vi "Smp_Data_transfer.vi"(0 "Connection ID":T1, 5 "SaveFilePath":path caption="Temp file path", 7 "Source file path":string, 9 "Read point":i32=256000, 11 "error in (no error)":errorcluster) -> (3 "Error Code":i16, 4 "Connection ID Out":T1, 6 "SaveFilePath.ref":path caption="Temp file path.ref", 10 "Stop":bool, 15 "error out":errorcluster)   [LabVIEW 2017]
uses:
  Driver/ConnectionID.ctl
  GL860_Driver.lvlib
panel:
  out "Progress bar":u8(slide) max=100 scale=0.0..100.0
  in  "Stop":bool
  # "Now transferring data..."
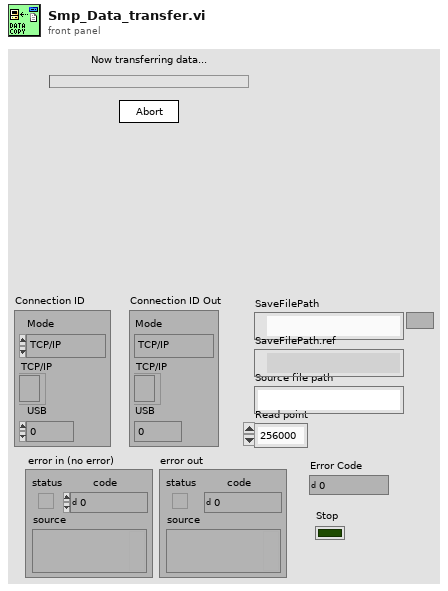
[diagram p1: front panel]
types:
  T1 = typedef "ConnectionID.ctl" = cluster{"Mode":enum16{"TCP/IP", "USB"}, "TCP/IP":refnum<k5>, "USB":i32}
  T2 = enum16{"open", "replace", "create", "open or create", "replace or create", "replace or create with confirmation"}
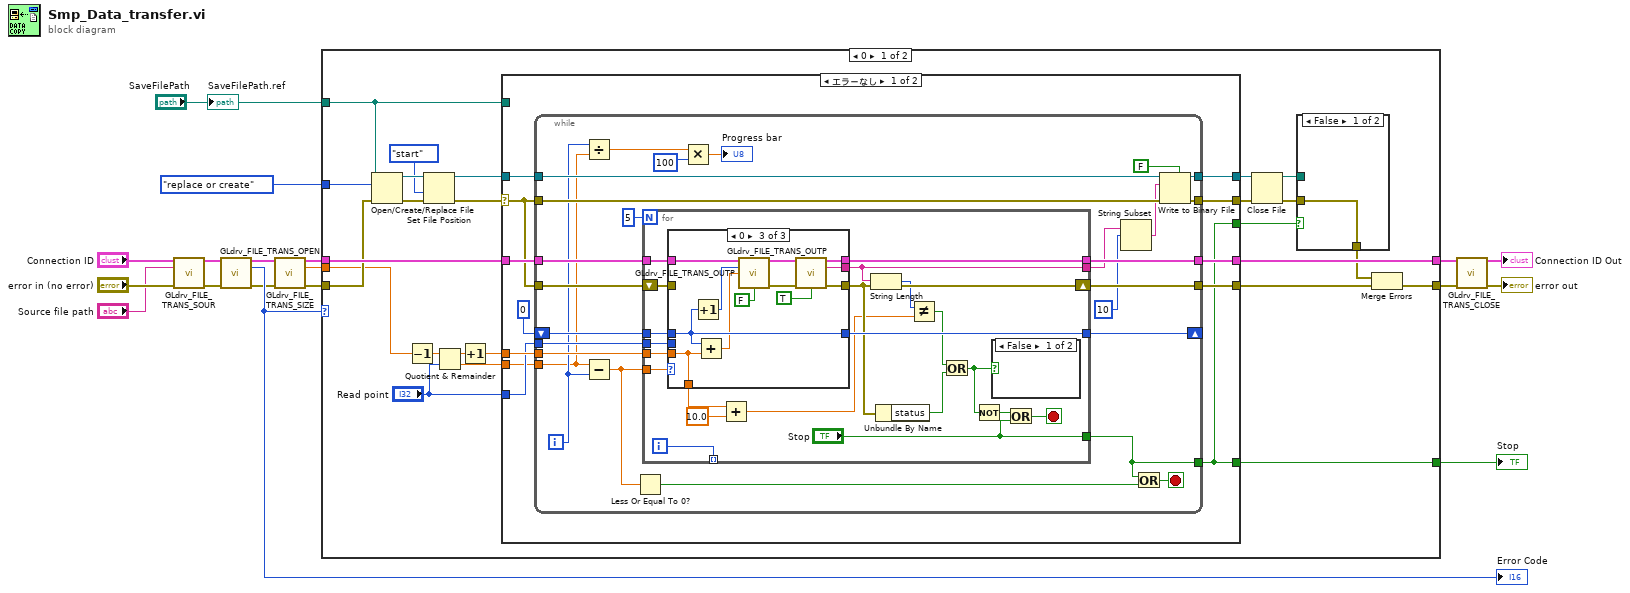
[diagram p0: block diagram]
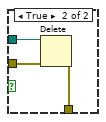
[diagram p2: hidden frame]
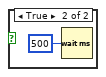
[diagram p3: hidden frame]
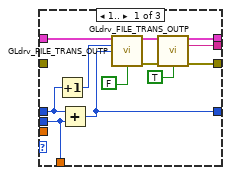
[diagram p4: hidden frame]
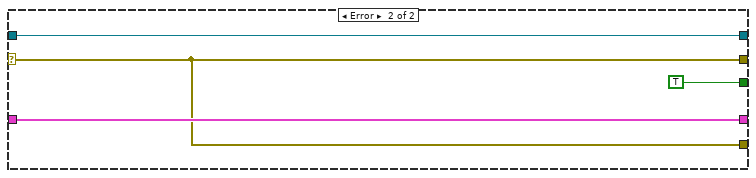
[diagram p6: hidden frame]
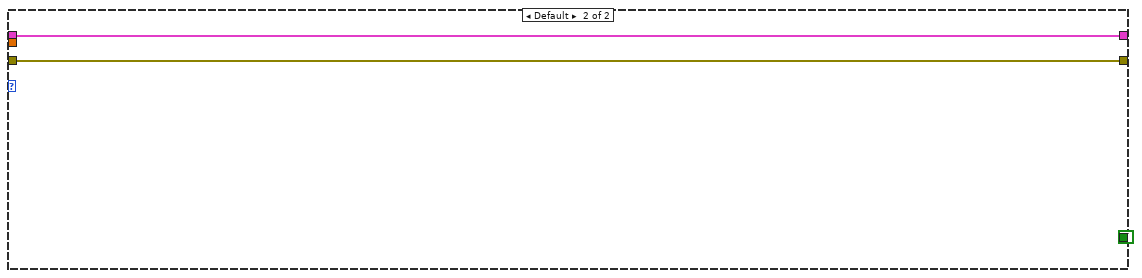
[diagram p7: hidden frame]
diagram:
  n1 = call "GLdrv_FILE_TRANS_SOUR.vi"("Connection ID"="Connection ID", "File Path"="Source file path", "error in (no error)"="error in (no error)") -> ("Connection ID Out"=w8:T1, "error out"=w7:errorcluster)  [unwired: 1 in, 10 out]
  n2 = call "GLdrv_FILE_TRANS_OPEN.vi"("Connection ID"=w8, "error in (no error)"=w7) -> ("Connection ID Out"=w5:T1, "Error Code"=w6:i16, "error out"=w4:errorcluster)  [unwired: 11 out]
  "Error Code" <- w6
  n3 = call "GLdrv_FILE_TRANS_SIZE.vi"("Connection ID"=w5, "error in (no error)"=w4) -> ("Connection ID Out"=w3:T1, "Size out"=w1:dbl, "error out"=w2:errorcluster)  [unwired: 11 out]
  n4 = case shown="0" w6 {
    tunnel: w3 -> [w40 w140]
    tunnel: w2 -> [w38 w141]
    tunnel: [w37 w140] -> w12
    tunnel: [w35 w141] -> w11
    tunnel: [w30 TRUE ("Stop")] -> w18
    tunnel: "SaveFilePath" -> [w27 _]
    tunnel: T2."replace or create" ("operation (0:open)") -> [w26 _]
    tunnel: w1 -> [w23 _]
    frame 0 {
      n5 = Open/Create/Replace File(file path (use dialog)=w27, error in=w38, operation (0:open)=w26) -> (refnum out=w42:refnum<file>, error out=w43:errorcluster)  [unwired: 4 out]
      n6 = Decrement(x=w23) -> (x-1=w29:dbl)
      n7 = Set File Position(refnum=w42, from (0:start)=enum16{"start", "end", "current"}."start" ("pos mode (0:2)"), error in=w43) -> (refnum out=w25:refnum<file>, error out=w24:errorcluster)  [unwired: 1 out]
      n8 = Quotient & Remainder(x=w29, y="Read point") -> (x-y*floor(x/y)=w32:dbl, floor(x/y)=w31:dbl)
      n9 = Increment(x=w32) -> (x+1=w28:dbl)
      n10 = case shown="エラーなし" w24 {
        selector: w24 -> [w53 w137]
        tunnel: w25 -> [w59 w136]
        tunnel: w40 -> [w58 w138]
        tunnel: w28 -> [w56 _]
        tunnel: w31 -> [w54 _]
        tunnel: "Read point" -> [w55 _]
        tunnel: [w52 w138] -> w37
        tunnel: [w51 w137] -> w36
        tunnel: [w49 w137] -> w34
        tunnel: [w48 w136] -> w33
        tunnel: w27 -> [_ _]
        tunnel: [w50 _] -> w30
        tunnel: [w50 TRUE ("Stop")] -> w19
        frame No Error {
          n11 = while {
            tunnel: w59 -> [w79]
            tunnel: w53 -> [w80]
            tunnel: w58 -> [w85]
            tunnel: w54 -> [w69]
            tunnel: [w84] -> w52
            tunnel: [w83] -> w51
            shift-right: [w81] -> _
            shift-left: 0 -> [w82]
            tunnel: w56 -> [w76]
            tunnel: [w78] -> w48
            tunnel: [w77] -> w49
            tunnel: w55 -> [w75]
            tunnel: w53 -> [w74]
            tunnel: [w64] -> w50
            i -> [w70]
            stop <- w71 stop-if-true
            n12 = Divide(x=w70, y=w69) -> (x/y=w66:dbl)
            n13 = Subtract(x=w69, y=w70) -> (x-y=w73:dbl)
            n14 = Less Or Equal To 0?(x=w73) -> (x <= 0?=w72:bool)
            n15 = for {
              N: 5 -> [_]
              tunnel: w85 -> [w106]
              tunnel: [w105] -> w84
              tunnel: w82 -> [w104]
              tunnel: [w103] -> w81
              tunnel: [w94] -> w61
              tunnel: w76 -> [w102]
              tunnel: w75 -> [w101]
              tunnel: w73 -> [w99]
              tunnel: ["Stop"] -> w64
              shift-right: [w98] -> w83
              shift-left: w74 -> [w100]
              tunnel: [w86] -> _ mode=indexing
              i -> [w86]
              stop <- w96 stop-if-true
              n16 = case shown="0" w99 {
                tunnel: w106 -> [w113 w122 w133]
                tunnel: [w116 w122 w128] -> w105
                tunnel: [w115 w121 w127] -> w98
                tunnel: w104 -> [w119 w120 w134]
                tunnel: [w109 w120 w134] -> w103
                tunnel: [w114 _ w126] -> w94
                tunnel: w102 -> [_ _ w123]
                tunnel: w101 -> [w108 _ _]
                tunnel: w100 -> [_ w121 _]
                tunnel: [w108 _ w123] -> w93
                frame 1.. {
                  n17 = Increment(x=w119) -> (x+1=w110:i32)
                  n18 = Add(x=w119, y=w108) -> (x+y=w109:i32)
                  n19 = call "GLdrv_FILE_TRANS_OUTP.vi"("Connection ID"=w113, "Start Byte"=w110, "End Byte"=w109, "Query(f)"=FALSE) -> ("Connection ID Out"=w118:T1, "error out"=w117:errorcluster)  [unwired: 1 in, 9 out]
                  n20 = call "GLdrv_FILE_TRANS_OUTP.vi"("Connection ID"=w118, "error in (no error)"=w117, "Query(f)"=TRUE) -> ("Connection ID Out"=w116:T1, "Data out"=w114:string, "error out"=w115:errorcluster)  [unwired: 2 in, 8 out]
                }
                frame ..-1 {
                }
                frame 0 {
                  n21 = Increment(x=w134) -> (x+1=w132:i32)
                  n22 = Add(x=w134, y=w123) -> (x+y=w131:dbl)
                  n23 = call "GLdrv_FILE_TRANS_OUTP.vi"("Connection ID"=w133, "Start Byte"=w132, "End Byte"=w131, "Query(f)"=FALSE) -> ("Connection ID Out"=w130:T1, "error out"=w129:errorcluster)  [unwired: 1 in, 9 out]
                  n24 = call "GLdrv_FILE_TRANS_OUTP.vi"("Connection ID"=w130, "error in (no error)"=w129, "Query(f)"=TRUE) -> ("Connection ID Out"=w128:T1, "Data out"=w126:string, "error out"=w127:errorcluster)  [unwired: 2 in, 8 out]
                }
              }
              n25 = Add(x=w93, y=10.0) -> (x+y=w90:dbl)
              n26 = String Length(string=w94) -> (length=w91:i32)
              n27 = Unbundle By Name(w98) -> ("status"=w88:bool)
              n28 = Not Equal?(x=w91, y=w90) -> (x != y?=w89:bool)
              n29 = Or(x=w89, y=w88) -> (x .or. y?=w87:bool)
              n30 = Not(x=w87) -> (.not. x?=w95:bool)
              n31 = case shown="FALSE" w87 {
                frame False {
                }
                frame True {
                  n32 = Wait (ms)(milliseconds to wait=u32 500) -> ()  [unwired: 1 out]
                }
              }
              n33 = Or(x=w95, y="Stop") -> (x .or. y?=w96:bool)
            }
            n34 = Multiply(x=w66, y=u8 100) -> (x*y=→"Progress bar":dbl)
            n35 = String Subset(string=w61, offset (0)=10 ("オフセット（0）")) -> (substring=w60:string)  [unwired: 1 in]
            n36 = Or(x=w64, y=w72) -> (x .or. y?=w71:bool)
            n37 = Write to Binary File(file (use dialog)=w79, data=w60, error in=w80, 5:FALSE ("prepend array or string size? (T)")) -> (refnum out=w78:refnum<file>, error out=w77:errorcluster)  [unwired: 3 out]
          }
        }
        frame Error {
        }
      }
      n38 = Close File(refnum=w33, error in=w34) -> (path=w20:path, error out=w22:errorcluster)
      n39 = case shown="FALSE" w19 {
        tunnel: w22 -> [w44 w47]
        tunnel: [w44 w46] -> w21
        tunnel: w20 -> [_ w45]
        frame False {
        }
        frame True {
          n40 = Delete(path (use dialog)=w45, error in=w47) -> (error out=w46:errorcluster)  [unwired: 5 out]
        }
      }
      n41 = Merge Errors(w21, w36) -> (w35:errorcluster)
    }
    frame Default {
    }
  }
  "Stop" <- w18
  n42 = call "GLdrv_FILE_TRANS_CLOSE.vi"("Connection ID"=w12, "error in (no error)"=w11) -> ("Connection ID Out"=→"Connection ID Out":T1, "error out"=→"error out":errorcluster)  [unwired: 12 out]
  "SaveFilePath.ref" <- "SaveFilePath"
